vi "Do Fire.vi"(9 "Height":i32, 10 "Width":i32, 11 "Pixel Array In":i32[](array[numeric])) -> (3 "Pixel Array Out":i32[](array[numeric]))   [LabVIEW 2018]
doc: "This is the main fire processing routine. It loops through every pixel of the pixel array except the bottom row (the fire source), and applies the Spread Fire logic."
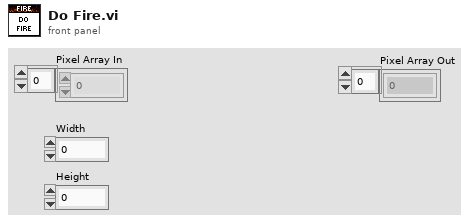
[diagram p1: front panel]
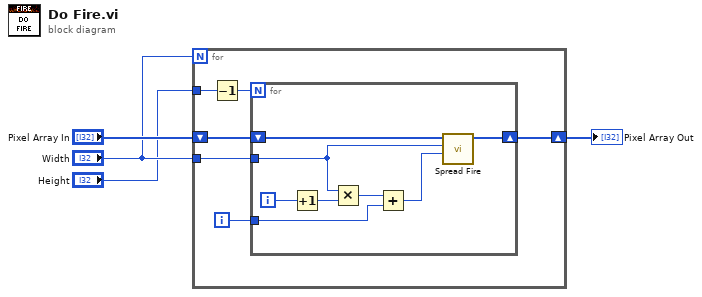
[diagram p0: block diagram]
diagram:
  n1 = for {
    N: "Width" -> [_]
    shift-right: [w8] -> w3
    shift-left: "Pixel Array In" -> [w9]
    tunnel: "Height" -> [w7]
    tunnel: "Width" -> [w5]
    i -> [w10]
    n2 = Decrement(x=w7) -> (x-1=w6:i32)
    n3 = for {
      N: w6 -> [_]
      tunnel: w10 -> [w15]
      shift-right: [w12] -> w8
      shift-left: w9 -> [w14]
      tunnel: w5 -> [w11]
      i -> [w18]
      n4 = Increment(x=w18) -> (x+1=w17:i32)
      n5 = Multiply(x=w11, y=w17) -> (x*y=w16:i32)
      n6 = Add(x=w16, y=w15) -> (x+y=w13:i32)
      n7 = call "Spread Fire.vi"("Pixel Source"=w13, "Width"=w11, "Pixel Array In"=w14) -> ("Pixel Array Out"=w12:i32[])  [unwired: 8 in]
    }
  }
  "Pixel Array Out" <- w3
